vi "VCI Read CAN Status.vi"(7 "pCANStatus":T1, 9 "CANIndex":u32, 10 "DevIndex":u32, 11 "DevType":u32) -> (3 "function return":u32, 5 "pCANStatus out":T1)   [LabVIEW 2010, in "ControlCAN.lvlib"]
doc: "unsigned int WINAPI VCI_ReadCANStatus(unsigned int DevType,unsigned int DevIndex,unsigned int CANIndex,PVCI_CAN_STATUS pCANStatus);"
uses:
  ControlCAN.lvlib
  ControlCAN/Ginkgo_Driver.dll
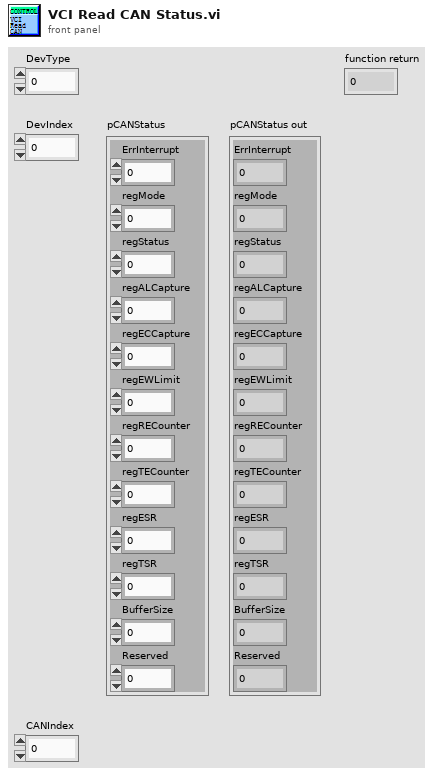
[diagram p1: front panel]
types:
  T1 = cluster{"ErrInterrupt":u8, "regMode":u8, "regStatus":u8, "regALCapture":u8, "regECCapture":u8, "regEWLimit":u8, "regRECounter":u8, "regTECounter":u8, "regESR":u32, "regTSR":u32, "BufferSize":u32, "Reserved":u32}
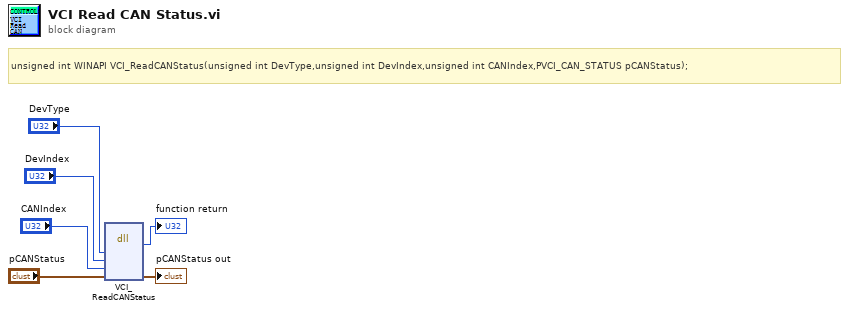
[diagram p0: block diagram]
diagram:
  # "unsigned int WINAPI VCI_ReadCANStatus(unsigned int DevType,unsigned int DevIndex,unsigned int CANIndex,PVCI_CAN_STATUS pCANStatus);"
  n1 = dll-call lib="E:/Project/vt_ginkgo/truck/Ginkgo Driver/vs2010/Ginkgo_USB-I2C&SPI&CAN_API_v2.0.3.3/lib/labview_32bit/ControlCAN/Ginkgo_Driver.*" fn="VCI_ReadCANStatus"("DevType"="DevType", "DevIndex"="DevIndex", "CANIndex"="CANIndex", "pCANStatus"="pCANStatus") -> (→"function return":u32, "pCANStatus"=→"pCANStatus out":T1)  [unwired: 6 in, 2 out]
